vi "Finish.vi"   [LabVIEW 2011]
doc: "This VI is called just before exiting. It is expected to close I/O refnum, save collected data, etc."
uses:
  Shared/Shifter State.ctl
  Apendage State.ctl
types:
  T1 = typedef "WPI_DigitalInputDevRef.ctl" = cluster{"DevStatus":errorcluster, "DIO Channel":T2, "Digital Module":T3}
  T2 = typedef "FPGA_DIOChannel.ctl" = enum8{"DIO 1", "DIO 2", "DIO 3", "DIO 4", "DIO 5", "DIO 6", "DIO 7", "DIO 8", "DIO 9", "DIO 10", "DIO 11", "DIO 12", "DIO 13", "DIO 14", "Invalid"}
  T3 = typedef "FPGA_TypedefDigitalModule.ctl" = enum16{"Digital Module 1", "Digital Module 2"}
  T4 = typedef "Apendage State.ctl" = enum16{"Unknown", "Down", "Up"}
  T5 = typedef "Shifter State.ctl" = enum16{"Unknown", "Low", "High"}
  T6 = typedef "WPI_CameraDevRef.ctl" = cluster{"Camera Address":string, "CameraStatus":errorcluster, "Acquire Image Notifier":refnum<notifier>}
  T7 = typedef "WPI_SolenoidDevRef.ctl" = cluster{"DevStatus":errorcluster, "Solenoid Module":T8, "Forward Solenoid Channel":T9, "Reverse Solenoid Channel":T9}
  T8 = typedef "FPGA_TypedefSolenoidModule.ctl" = enum16{"Solenoid Module 1", "Solenoid Module 2"}
  T9 = typedef "WPI_SolenoidChannel.ctl" = enum8{"Solenoid 1", "Solenoid 2", "Solenoid 3", "Solenoid 4", "Solenoid 5", "Solenoid 6", "Solenoid 7", "Solenoid 8", "Invalid"}
  T10 = typedef "WPI_RelayDevRef.ctl" = cluster{"DevStatus":errorcluster, "Relay Channel":T11, "Digital Module":T3, "Relay Direction":T12}
  T11 = typedef "FPGA_DIORelayChannel.ctl" = enum8{"Relay 1", "Relay 2", "Relay 3", "Relay 4", "Relay 5", "Relay 6", "Relay 7", "Relay 8", "Invalid"}
  T12 = typedef "WPI_RelayDirection.ctl" = enum16{"Both directions", "Forward only", "Reverse only"}
  T13 = typedef "WPI_GyroDevRef.ctl" = cluster{"DevStatus":errorcluster, "Analog Module":T14, "Analog Channel":T15, "Offset":dbl, "Gain (VoltsPerDegree/Second)":dbl}
  T14 = typedef "FPGA_TypedefAnalogModule.ctl" = enum16{"Analog Module 1", "Analog Module 2"}
  T15 = typedef "FPGA_AIChannel.ctl" = enum8{"AI 1", "AI 2", "AI 3", "AI 4", "AI 5", "AI 6", "AI 7", "AI 8", "Invalid"}
  T16 = typedef "WPI_AnalogChannelDevRef.ctl" = cluster{"DevStatus":errorcluster, "Analog Module":T14, "Analog Channel":T15}
  T17 = typedef "WPI_MotorControlDeviceRef.ctl" = cluster{"DeviceStatus":errorcluster, "Type":enum16{"PWM", "CAN"}, "PWM":cluster{"Digital Module":T3, "PWM Channel":T18, "DeadBand":T19}, "CAN":cluster{"Device Number":u8, "Control Mode":T20, "Semaphore":T21, "Max Vout":dbl}, "Invert":bool, "TransformRef":T22, "InvTransformRef":T22}
  T18 = typedef "FPGA_DIOPWMChannel.ctl" = enum8{"PWM 1", "PWM 2", "PWM 3", "PWM 4", "PWM 5", "PWM 6", "PWM 7", "PWM 8", "PWM 9", "PWM 10", "Invalid"}
  T19 = typedef "WPI_PWMDeadband.ctl" = cluster{"Name":string, "maxPositivePwm":i32, "minPositivePwm":i32, "centerPwm":i32, "maxNegativePwm":i32, "minNegativePwm":i32, "angularRange":u16}
  T20 = typedef "WPI_CANJaguar_ControlMode.ctl" = enum8{"Percent VBus", "Current", "Speed", "Position", "Voltage"}
  T21 = typedef "Semaphore RefNum" = refnum<k1>
  T22 = typedef "WPI_PWMTransform_ConPane.ctl" = refnum<vi>
  T23 = typedef "WPI_JoystickDevRef.ctl" = cluster{"Device":T24}
  T24 = typedef "WPI_JoystickDeviceEnum.ctl" = enum16{"USB 1", "USB 2", "USB 3", "USB 4", "Kinect 1", "Kinect 2"}
  T25 = typedef "WPI_RobotDriveDevRef.ctl" = cluster{"DevStatus":errorcluster, "Motors[]":T17[], "Square Inputs":bool, "Max Output":dbl, "Isochronous":bool}
  T26 = typedef "WPI_CounterDevRef.ctl" = cluster{"DevStatus":errorcluster, "CntIndex":T27}
  T27 = typedef "FPGA_CounterCtrSystemIndex.ctl" = enum8{"Ctr 0", "Ctr 1", "Ctr 2", "Ctr 3", "Ctr 4", "Ctr 5", "Ctr 6", "Ctr 7", "Invalid"}
  T28 = typedef "WPI_EncoderDevRef.ctl" = cluster{"DevStatus":errorcluster, "EncoderIndex":T29, "CounterIndex":T27, "DistancePerCount":dbl, "Decoding Type":T30}
  T29 = typedef "FPGA_EncoderIdx.ctl" = enum8{"Enc 0", "Enc 1", "Enc 2", "Enc 3", "Invalid"}
  T30 = typedef "WPI_EncoderType.ctl" = enum16{"1x", "2x", "4x"}
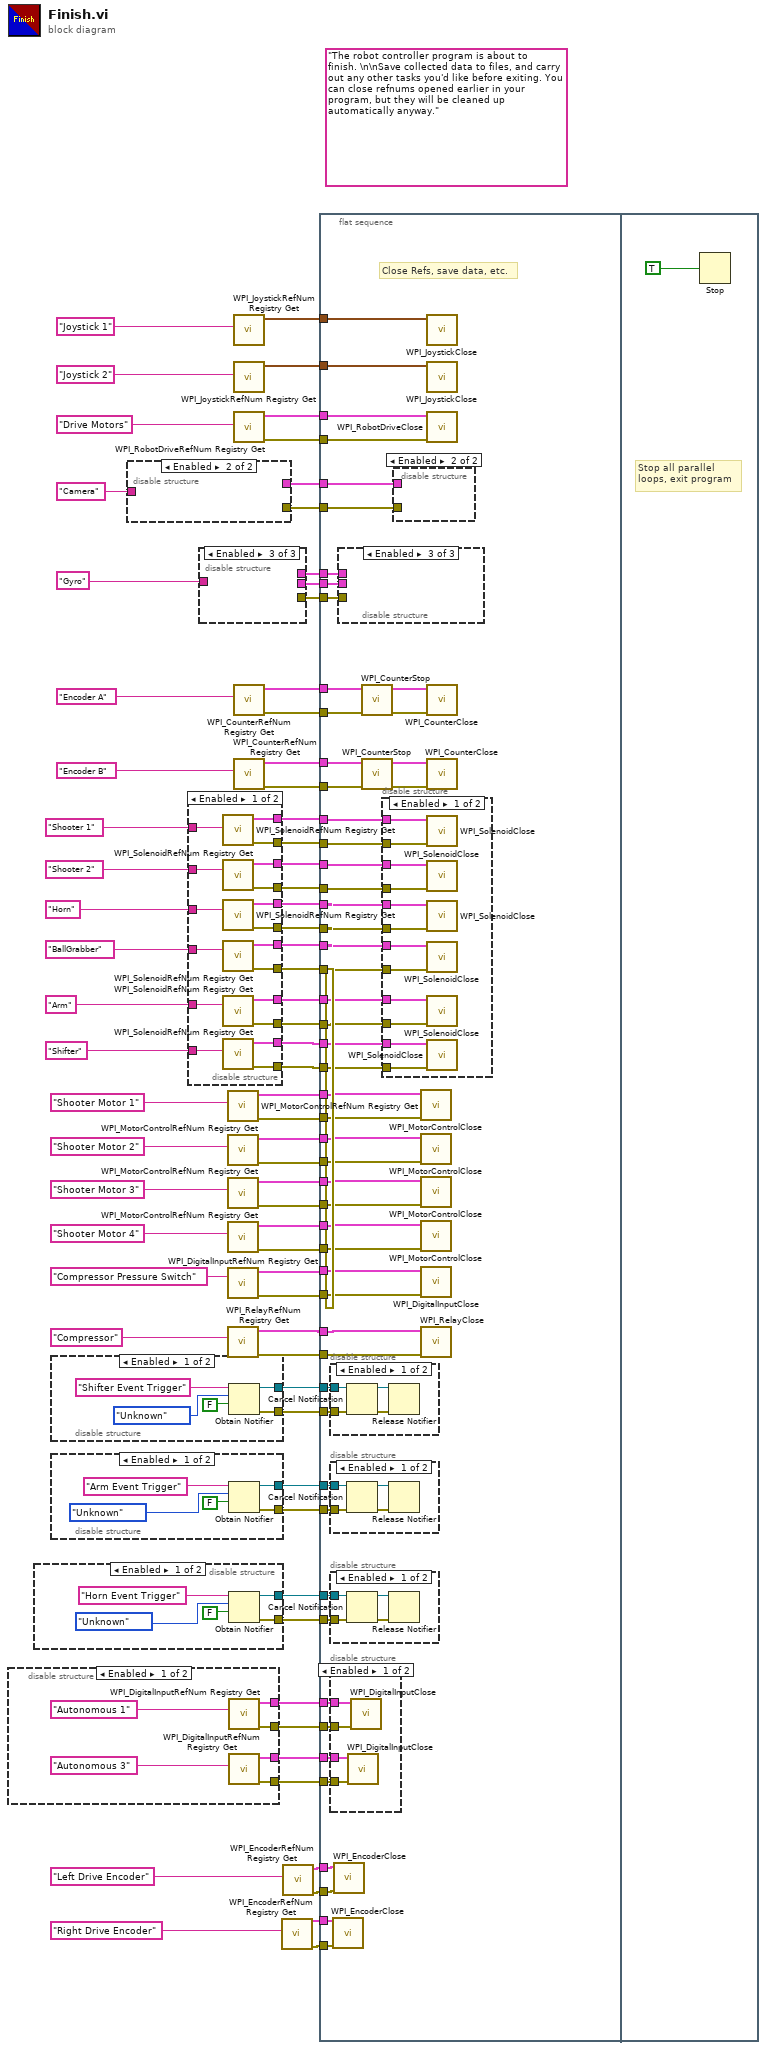
[diagram p0: block diagram]
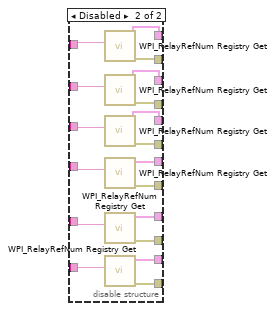
[diagram p3: hidden frame]
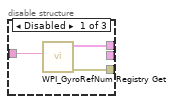
[diagram p7: hidden frame]
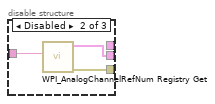
[diagram p8: hidden frame]
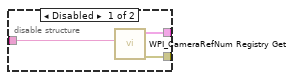
[diagram p9: hidden frame]
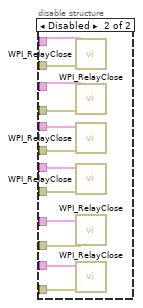
[diagram p11: hidden frame]
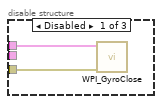
[diagram p15: hidden frame]
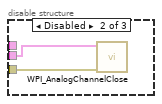
[diagram p16: hidden frame]
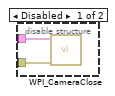
[diagram p17: hidden frame]
diagram:
  (unwired) "The robot controller program is about to finish. \n\nSave collected data to files, and carry out any other tasks you'd like before exiting. You can close refnums opened earlier in your program, but they will be cleaned up automatically anyway."
  n1 = disable-structure shown="Enabled" {
    disable-tunnel: [w78 _] -> w10
    disable-tunnel: [w77 _] -> w9
    disable-tunnel: [w76 _] -> w8
    disable-tunnel: [w75 _] -> w7
    frame Enabled {
      n2 = call <vilib>:"WPI_DigitalInputRefNum Registry Get.vi"("refnum name"="Autonomous 1") -> ("error out"=w78:errorcluster, "DigitalInputDevRef"=w77:T1)  [unwired: 9 in]
      n3 = call <vilib>:"WPI_DigitalInputRefNum Registry Get.vi"("refnum name"="Autonomous 3") -> ("error out"=w76:errorcluster, "DigitalInputDevRef"=w75:T1)  [unwired: 9 in]
    }
    frame Disabled {
    }
  }
  n4 = disable-structure shown="Enabled" {
    disable-tunnel: [w82 _] -> w12
    disable-tunnel: [w81 _] -> w11
    frame Enabled {
      n5 = Obtain Notifier(name (unnamed)="Horn Event Trigger", notification data type=Apendage_State."Unknown", create if not found? (T)=FALSE) -> (notifier out=w82:refnum<notifier>, error out=w81:errorcluster)  [unwired: 1 in, 1 out]
    }
    frame Disabled {
    }
  }
  n6 = disable-structure shown="Enabled" {
    disable-tunnel: [w85 _] -> w16
    disable-tunnel: [w84 _] -> w15
    frame Enabled {
      n7 = Obtain Notifier(name (unnamed)="Shifter Event Trigger", notification data type=Shifter_State."Unknown", create if not found? (T)=FALSE) -> (notifier out=w85:refnum<notifier>, error out=w84:errorcluster)  [unwired: 1 in, 1 out]
    }
    frame Disabled {
    }
  }
  n8 = disable-structure shown="Enabled" {
    disable-tunnel: [w92 _] -> w13
    disable-tunnel: [w91 _] -> w14
    frame Enabled {
      n9 = Obtain Notifier(name (unnamed)="Arm Event Trigger", notification data type=Apendage_State."Unknown", create if not found? (T)=FALSE) -> (notifier out=w92:refnum<notifier>, error out=w91:errorcluster)  [unwired: 1 in, 1 out]
    }
    frame Disabled {
    }
  }
  n10 = disable-structure shown="Enabled" {
    disable-tunnel: [w96 _] -> w69
    disable-tunnel: [w95 _] -> w65
    disable-tunnel: "Camera" ("refnum name") -> [w94 _]
    frame Disabled {
      n11 = call <vilib>:"WPI_CameraRefNum Registry Get.vi"("refnum name"=w94) -> ("error out"=w95:errorcluster, "CameraDevRef"=w96:T6)  [unwired: 1 in, 8 out]
    }
    frame Enabled {
    }
  }
  n12 = disable-structure shown="Enabled" {
    disable-tunnel: [w114 w127] -> w63
    disable-tunnel: [w113 w126] -> w62
    disable-tunnel: "Shifter" ("refnum name") -> [w112 w115]
    disable-tunnel: [w111 w121] -> w54
    disable-tunnel: [w110 w132] -> w53
    disable-tunnel: [w109 w131] -> w52
    disable-tunnel: [w108 w122] -> w51
    disable-tunnel: "Shooter 1" ("refnum name") -> [w107 w120]
    disable-tunnel: "Shooter 2" ("refnum name") -> [w106 w119]
    disable-tunnel: [w105 w123] -> w30
    disable-tunnel: [w104 w130] -> w29
    disable-tunnel: [w103 w129] -> w28
    disable-tunnel: [w102 w124] -> w27
    disable-tunnel: [w101 w125] -> w26
    disable-tunnel: [w100 w128] -> w25
    disable-tunnel: "Horn" ("refnum name") -> [w99 w118]
    disable-tunnel: "BallGrabber" ("refnum name") -> [w98 w117]
    disable-tunnel: "Arm" ("refnum name") -> [w97 w116]
    frame Enabled {
      n13 = call <vilib>:"WPI_SolenoidRefNum Registry Get.vi"("refnum name"=w107) -> ("error out"=w110:errorcluster, "SolenoidDevRef"=w111:T7)  [unwired: 9 in]
      n14 = call <vilib>:"WPI_SolenoidRefNum Registry Get.vi"("refnum name"=w106) -> ("error out"=w109:errorcluster, "SolenoidDevRef"=w108:T7)  [unwired: 9 in]
      n15 = call <vilib>:"WPI_SolenoidRefNum Registry Get.vi"("refnum name"=w99) -> ("error out"=w104:errorcluster, "SolenoidDevRef"=w105:T7)  [unwired: 9 in]
      n16 = call <vilib>:"WPI_SolenoidRefNum Registry Get.vi"("refnum name"=w98) -> ("error out"=w103:errorcluster, "SolenoidDevRef"=w102:T7)  [unwired: 9 in]
      n17 = call <vilib>:"WPI_SolenoidRefNum Registry Get.vi"("refnum name"=w97) -> ("error out"=w100:errorcluster, "SolenoidDevRef"=w101:T7)  [unwired: 9 in]
      n18 = call <vilib>:"WPI_SolenoidRefNum Registry Get.vi"("refnum name"=w112) -> ("error out"=w114:errorcluster, "SolenoidDevRef"=w113:T7)  [unwired: 9 in]
    }
    frame Disabled {
      n19 = call <vilib>:"WPI_RelayRefNum Registry Get.vi"("refnum name"=w120) -> ("error out"=w132:errorcluster, "RelayDevRef"=w121:T10)  [unwired: 9 in]
      n20 = call <vilib>:"WPI_RelayRefNum Registry Get.vi"("refnum name"=w119) -> ("error out"=w131:errorcluster, "RelayDevRef"=w122:T10)  [unwired: 9 in]
      n21 = call <vilib>:"WPI_RelayRefNum Registry Get.vi"("refnum name"=w118) -> ("error out"=w130:errorcluster, "RelayDevRef"=w123:T10)  [unwired: 9 in]
      n22 = call <vilib>:"WPI_RelayRefNum Registry Get.vi"("refnum name"=w117) -> ("error out"=w129:errorcluster, "RelayDevRef"=w124:T10)  [unwired: 9 in]
      n23 = call <vilib>:"WPI_RelayRefNum Registry Get.vi"("refnum name"=w116) -> ("error out"=w128:errorcluster, "RelayDevRef"=w125:T10)  [unwired: 9 in]
      n24 = call <vilib>:"WPI_RelayRefNum Registry Get.vi"("refnum name"=w115) -> ("error out"=w127:errorcluster, "RelayDevRef"=w126:T10)  [unwired: 9 in]
    }
  }
  n25 = disable-structure shown="Enabled" {
    disable-tunnel: [w135 w138 _] -> w21
    disable-tunnel: [w134 _ _] -> w20
    disable-tunnel: [_ w137 _] -> w19
    disable-tunnel: "Gyro" ("refnum name") -> [w133 w136 _]
    frame Disabled {
      n26 = call <vilib>:"WPI_GyroRefNum Registry Get.vi"("refnum name"=w133) -> ("error out"=w135:errorcluster, "GyroDevRef"=w134:T13)  [unwired: 9 in]
    }
    frame Disabled {
      n27 = call <vilib>:"WPI_AnalogChannelRefNum Registry Get.vi"("refnum name"=w136) -> ("error out"=w138:errorcluster, "AIDeviceRef"=w137:T16)  [unwired: 9 in]
    }
    frame Enabled {
    }
  }
  n28 = call <vilib>:"WPI_MotorControlRefNum Registry Get.vi"("refnum name"="Shooter Motor 1") -> ("error out"=w48:errorcluster, "MotorControlDevRef"=w47:T17)  [unwired: 9 in]
  n29 = call <vilib>:"WPI_MotorControlRefNum Registry Get.vi"("refnum name"="Shooter Motor 2") -> ("error out"=w45:errorcluster, "MotorControlDevRef"=w46:T17)  [unwired: 9 in]
  n30 = call <vilib>:"WPI_MotorControlRefNum Registry Get.vi"("refnum name"="Shooter Motor 3") -> ("error out"=w44:errorcluster, "MotorControlDevRef"=w43:T17)  [unwired: 9 in]
  n31 = call <vilib>:"WPI_MotorControlRefNum Registry Get.vi"("refnum name"="Shooter Motor 4") -> ("error out"=w41:errorcluster, "MotorControlDevRef"=w42:T17)  [unwired: 9 in]
  n32 = call <vilib>:"WPI_DigitalInputRefNum Registry Get.vi"("refnum name"="Compressor Pressure Switch") -> ("error out"=w36:errorcluster, "DigitalInputDevRef"=w35:T1)  [unwired: 9 in]
  n33 = call <vilib>:"WPI_RelayRefNum Registry Get.vi"("refnum name"="Compressor") -> ("error out"=w33:errorcluster, "RelayDevRef"=w32:T10)  [unwired: 9 in]
  n34 = call <vilib>:"WPI_JoystickRefNum Registry Get.vi"("refnum name"="Joystick 1") -> ("JoystickDevRef"=w70:T23)  [unwired: 1 in, 9 out]
  n35 = call <vilib>:"WPI_JoystickRefNum Registry Get.vi"("refnum name"="Joystick 2") -> ("JoystickDevRef"=w67:T23)  [unwired: 1 in, 9 out]
  n36 = call <vilib>:"WPI_RobotDriveRefNum Registry Get.vi"("refnum name"="Drive Motors") -> ("error out"=w64:errorcluster, "RobotDriveDevRef"=w71:T25)  [unwired: 1 in, 8 out]
  n37 = call <vilib>:"WPI_CounterRefNum Registry Get.vi"("refnum name"="Encoder A") -> ("error out"=w60:errorcluster, "CounterDevRef"=w59:T26)  [unwired: 9 in]
  n38 = call <vilib>:"WPI_CounterRefNum Registry Get.vi"("refnum name"="Encoder B") -> ("error out"=w57:errorcluster, "CounterDevRef"=w58:T26)  [unwired: 9 in]
  n39 = call <vilib>:"WPI_EncoderRefNum Registry Get.vi"("refnum name"="Right Drive Encoder") -> ("error out"=w4:errorcluster, "EncoderDevRef"=w3:T28)  [unwired: 9 in]
  n40 = call <vilib>:"WPI_EncoderRefNum Registry Get.vi"("refnum name"="Left Drive Encoder") -> ("error out"=w6:errorcluster, "EncoderDevRef"=w5:T28)  [unwired: 9 in]
  n41 = flat-sequence {
    tunnel: w71 -> [w193]
    tunnel: w70 -> [w192]
    tunnel: w69 -> [w191]
    tunnel: w67 -> [w190]
    tunnel: w65 -> [w189]
    tunnel: w64 -> [w188]
    tunnel: w63 -> [w187]
    tunnel: w62 -> [w186]
    tunnel: w60 -> [w185]
    tunnel: w59 -> [w184]
    tunnel: w57 -> [w178]
    tunnel: w58 -> [w179]
    tunnel: w53 -> [w176]
    tunnel: w54 -> [w177]
    tunnel: w52 -> [w175]
    tunnel: w51 -> [w174]
    tunnel: w48 -> [w173]
    tunnel: w47 -> [w172]
    tunnel: w45 -> [w170]
    tunnel: w46 -> [w171]
    tunnel: w44 -> [w169]
    tunnel: w43 -> [w168]
    tunnel: w41 -> [w166]
    tunnel: w42 -> [w167]
    tunnel: w36 -> [w165]
    tunnel: w35 -> [w164]
    tunnel: w33 -> [w163]
    tunnel: w32 -> [w162]
    tunnel: w29 -> [w160]
    tunnel: w30 -> [w161]
    tunnel: w28 -> [w159]
    tunnel: w27 -> [w158]
    tunnel: w25 -> [w156]
    tunnel: w26 -> [w157]
    tunnel: w21 -> [w155]
    tunnel: w20 -> [w154]
    tunnel: w19 -> [w153]
    tunnel: w16 -> [w152]
    tunnel: w15 -> [w151]
    tunnel: w13 -> [w149]
    tunnel: w14 -> [w150]
    tunnel: w12 -> [w148]
    tunnel: w11 -> [w147]
    tunnel: w10 -> [w146]
    tunnel: w9 -> [w145]
    tunnel: w8 -> [w144]
    tunnel: w7 -> [w143]
    tunnel: w6 -> [w142]
    tunnel: w5 -> [w141]
    tunnel: w4 -> [w140]
    tunnel: w3 -> [w139]
    frame #0 {
      # "Close Refs, save data, etc."
      n42 = disable-structure shown="Enabled" {
        disable-tunnel: w152 -> [w233 _]
        disable-tunnel: w151 -> [w232 _]
        frame Enabled {
          n43 = Cancel Notification(0:w233, 3:w232) -> (8:w231:refnum<notifier>, 11:w230:errorcluster)  [unwired: 1 out]
          n44 = Release Notifier(notifier=w231, error in (no error)=w230) -> ()  [unwired: 1 in, 3 out]
        }
        frame Disabled {
        }
      }
      n45 = disable-structure shown="Enabled" {
        disable-tunnel: w149 -> [w229 _]
        disable-tunnel: w150 -> [w228 _]
        frame Enabled {
          n46 = Cancel Notification(0:w229, 3:w228) -> (8:w227:refnum<notifier>, 11:w226:errorcluster)  [unwired: 1 out]
          n47 = Release Notifier(notifier=w227, error in (no error)=w226) -> ()  [unwired: 1 in, 3 out]
        }
        frame Disabled {
        }
      }
      n48 = disable-structure shown="Enabled" {
        disable-tunnel: w148 -> [w225 _]
        disable-tunnel: w147 -> [w224 _]
        frame Enabled {
          n49 = Cancel Notification(0:w225, 3:w224) -> (8:w223:refnum<notifier>, 11:w222:errorcluster)  [unwired: 1 out]
          n50 = Release Notifier(notifier=w223, error in (no error)=w222) -> ()  [unwired: 1 in, 3 out]
        }
        frame Disabled {
        }
      }
      n51 = disable-structure shown="Enabled" {
        disable-tunnel: w146 -> [w197 _]
        disable-tunnel: w145 -> [w196 _]
        disable-tunnel: w144 -> [w195 _]
        disable-tunnel: w143 -> [w194 _]
        frame Enabled {
          n52 = call <vilib>:"WPI_DigitalInputClose.vi"("error in (no error)"=w195, "DigitalInputDevRef"=w194) -> ()  [unwired: 9 in, 1 out]
          n53 = call <vilib>:"WPI_DigitalInputClose.vi"("error in (no error)"=w197, "DigitalInputDevRef"=w196) -> ()  [unwired: 9 in, 1 out]
        }
        frame Disabled {
        }
      }
      n54 = call <vilib>:"WPI_EncoderClose.vi"("error in (no error)"=w140, "EncoderDevRef"=w139) -> ()  [unwired: 1 in, 9 out]
      n55 = call <vilib>:"WPI_EncoderClose.vi"("error in (no error)"=w142, "EncoderDevRef"=w141) -> ()  [unwired: 1 in, 9 out]
      n56 = disable-structure shown="Enabled" {
        disable-tunnel: w155 -> [w235 w237 _]
        disable-tunnel: w154 -> [w234 _ _]
        disable-tunnel: w153 -> [_ w236 _]
        frame Disabled {
          n57 = call <vilib>:"WPI_GyroClose.vi"("error in (no error)"=w235, "GyroDevRef"=w234) -> ()  [unwired: 9 in, 1 out]
        }
        frame Disabled {
          n58 = call <vilib>:"WPI_AnalogChannelClose.vi"("error in (no error)"=w237, "AIDeviceRef"=w236) -> ()  [unwired: 9 in, 1 out]
        }
        frame Enabled {
        }
      }
      n59 = call <vilib>:"WPI_CounterStop.vi"("error in (no error)"=w185, "CounterDevRef in"=w184) -> ("error out"=w183:errorcluster, "CounterDevRef out"=w182:T26)  [unwired: 8 in]
      n60 = call <vilib>:"WPI_CounterStop.vi"("error in (no error)"=w178, "CounterDevRef in"=w179) -> ("error out"=w180:errorcluster, "CounterDevRef out"=w181:T26)  [unwired: 8 in]
      n61 = disable-structure shown="Enabled" {
        disable-tunnel: w187 -> [w209 w216]
        disable-tunnel: w186 -> [w208 w210]
        disable-tunnel: w177 -> [w207 w215]
        disable-tunnel: w176 -> [w206 w221]
        disable-tunnel: w175 -> [w205 w220]
        disable-tunnel: w174 -> [w204 w214]
        disable-tunnel: w161 -> [w203 w213]
        disable-tunnel: w160 -> [w202 w219]
        disable-tunnel: w159 -> [w201 w218]
        disable-tunnel: w158 -> [w200 w212]
        disable-tunnel: w157 -> [w199 w211]
        disable-tunnel: w156 -> [w198 w217]
        frame Enabled {
          n62 = call <vilib>:"WPI_SolenoidClose.vi"("error in (no error)"=w206, "SolenoidDevRef"=w207) -> ()  [unwired: 9 in, 1 out]
          n63 = call <vilib>:"WPI_SolenoidClose.vi"("error in (no error)"=w205, "SolenoidDevRef"=w204) -> ()  [unwired: 9 in, 1 out]
          n64 = call <vilib>:"WPI_SolenoidClose.vi"("error in (no error)"=w202, "SolenoidDevRef"=w203) -> ()  [unwired: 9 in, 1 out]
          n65 = call <vilib>:"WPI_SolenoidClose.vi"("error in (no error)"=w201, "SolenoidDevRef"=w200) -> ()  [unwired: 9 in, 1 out]
          n66 = call <vilib>:"WPI_SolenoidClose.vi"("error in (no error)"=w198, "SolenoidDevRef"=w199) -> ()  [unwired: 9 in, 1 out]
          n67 = call <vilib>:"WPI_SolenoidClose.vi"("error in (no error)"=w209, "SolenoidDevRef"=w208) -> ()  [unwired: 9 in, 1 out]
        }
        frame Disabled {
          n68 = call <vilib>:"WPI_RelayClose.vi"("error in (no error)"=w221, "RelayDevRef"=w215) -> ()  [unwired: 9 in, 1 out]
          n69 = call <vilib>:"WPI_RelayClose.vi"("error in (no error)"=w220, "RelayDevRef"=w214) -> ()  [unwired: 9 in, 1 out]
          n70 = call <vilib>:"WPI_RelayClose.vi"("error in (no error)"=w219, "RelayDevRef"=w213) -> ()  [unwired: 9 in, 1 out]
          n71 = call <vilib>:"WPI_RelayClose.vi"("error in (no error)"=w218, "RelayDevRef"=w212) -> ()  [unwired: 9 in, 1 out]
          n72 = call <vilib>:"WPI_RelayClose.vi"("error in (no error)"=w217, "RelayDevRef"=w211) -> ()  [unwired: 9 in, 1 out]
          n73 = call <vilib>:"WPI_RelayClose.vi"("error in (no error)"=w216, "RelayDevRef"=w210) -> ()  [unwired: 9 in, 1 out]
        }
      }
      n74 = disable-structure shown="Enabled" {
        disable-tunnel: w191 -> [w239 _]
        disable-tunnel: w189 -> [w238 _]
        frame Disabled {
          n75 = call <vilib>:"WPI_CameraClose.vi"("error in (no error)"=w238, "CameraDevRef"=w239) -> ()  [unwired: 10 out]
        }
        frame Enabled {
        }
      }
      n76 = call <vilib>:"WPI_MotorControlClose.vi"("error in (no error)"=w173, "MotorControlDevRef"=w172) -> ()  [unwired: 9 in, 1 out]
      n77 = call <vilib>:"WPI_MotorControlClose.vi"("error in (no error)"=w170, "MotorControlDevRef"=w171) -> ()  [unwired: 9 in, 1 out]
      n78 = call <vilib>:"WPI_MotorControlClose.vi"("error in (no error)"=w169, "MotorControlDevRef"=w168) -> ()  [unwired: 9 in, 1 out]
      n79 = call <vilib>:"WPI_MotorControlClose.vi"("error in (no error)"=w166, "MotorControlDevRef"=w167) -> ()  [unwired: 9 in, 1 out]
      n80 = call <vilib>:"WPI_DigitalInputClose.vi"("error in (no error)"=w165, "DigitalInputDevRef"=w164) -> ()  [unwired: 9 in, 1 out]
      n81 = call <vilib>:"WPI_RelayClose.vi"("error in (no error)"=w163, "RelayDevRef"=w162) -> ()  [unwired: 9 in, 1 out]
      n82 = call <vilib>:"WPI_JoystickClose.vi"("JoystickDevRef"=w192) -> ()  [unwired: 11 out]
      n83 = call <vilib>:"WPI_JoystickClose.vi"("JoystickDevRef"=w190) -> ()  [unwired: 11 out]
      n84 = call <vilib>:"WPI_RobotDriveClose.vi"("error in (no error)"=w188, "RobotDriveDevRef"=w193) -> ()  [unwired: 10 out]
      n85 = call <vilib>:"WPI_CounterClose.vi"("error in (no error)"=w183, "CounterDevRef"=w182) -> ()  [unwired: 9 in, 1 out]
      n86 = call <vilib>:"WPI_CounterClose.vi"("error in (no error)"=w180, "CounterDevRef"=w181) -> ()  [unwired: 9 in, 1 out]
    }
    frame #1 {
      # "Stop all parallel\nloops, exit program"
      n87 = Stop(stop? (T)=TRUE ("Quit")) -> ()
    }
  }
